vi "FRCts_ClientAPI_Build URL.vi"(8 "error in":errorcluster, 10 "Resource":string, 11 "Collection":T1) -> (0 "error out":errorcluster, 2 "URL":string)   [LabVIEW 2013, in "FRCts_ClientAPI.lvlib"]
doc: "This VI builds the URL that will be used to Post, Get, Put, or Delete a certain resource based on the specified collection and resource"
uses:
  FRCts_ClientAPI.lvlib
  FRCts_ClientAPI_Collection.ctl
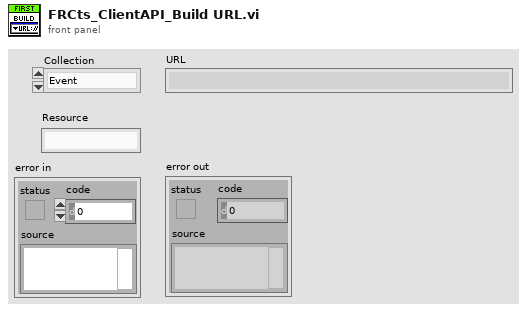
[diagram p1: front panel]
types:
  T1 = typedef "FRCts_ClientAPI.lvlib/FRCts_ClientAPI_Collection.ctl" = enum16{"Event", "Events", "Team", "Teams", "Request", "Requests", "Reports"}
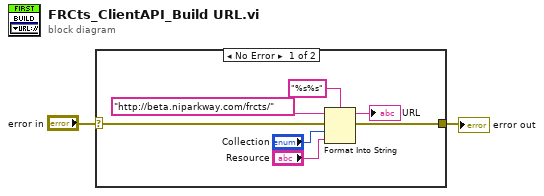
[diagram p0: block diagram]
diagram:
  n1 = case shown="No Error" "error in" {
    selector: "error in" -> [w4 w10]
    tunnel: [w3 w10] -> w2
    frame No Error {
      n2 = Format Into String(format string="%s%s", initial string="http://beta.niparkway.com/frcts/", error in=w4, "Collection", "Resource") -> (resulting string=→"URL":string, error out=w3:errorcluster)
    }
    frame Error {
    }
  }
  "error out" <- w2
